vi "SetParam.vi"(8 "error in (no error)":errorcluster caption="entrée d'erreur (pas d'erreur)", 10 "fbeta_score":T1={"beta"=0.0, "labels"=[], "pos_label"={"dtype_pos_label"="int", "pos_label"="1"}, "average"="binary", "sample_weight"=[], "zero_division"={"dtype_zero_division"="str", "zero_division"="warn"}}, 11 "Fbeta_Score.lvclass":refnum<class "Fbeta_Score.lvclass">) -> (0 "error out":errorcluster caption="sortie d'erreur", 3 "Fbeta_Score.lvclass":refnum<class "Fbeta_Score.lvclass">)   [LabVIEW 2020, in "Fbeta_Score.lvclass"]
doc: "Set Parameters"
uses:
  Fbeta_Score.lvclass
  Fbeta_Score.lvclass/Fbeta_Score.ctl
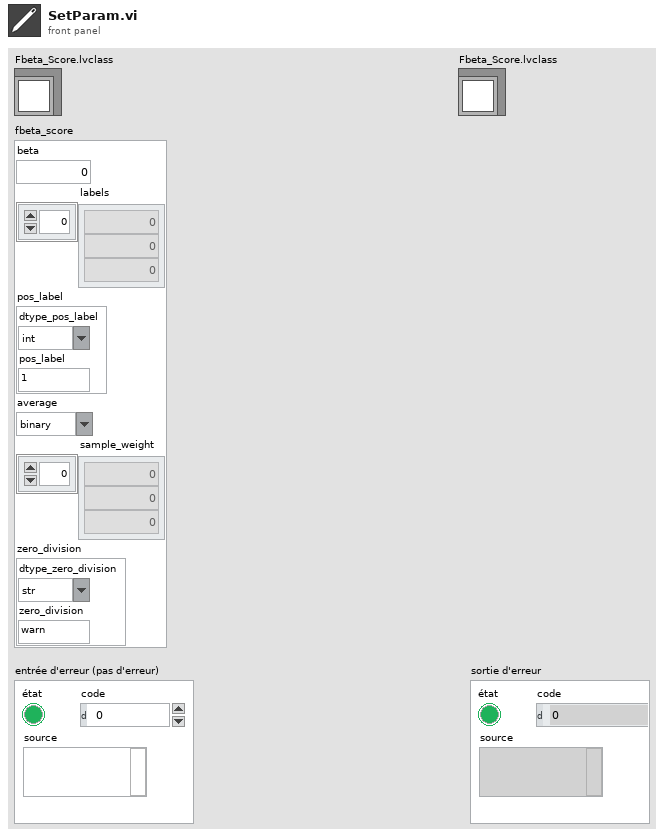
[diagram p1: front panel]
types:
  T1 = cluster{"beta":dbl, "labels":i32[], "pos_label":cluster{"dtype_pos_label":string, "pos_label":string}, "average":string, "sample_weight":dbl[], "zero_division":cluster{"dtype_zero_division":string, "zero_division":string}}
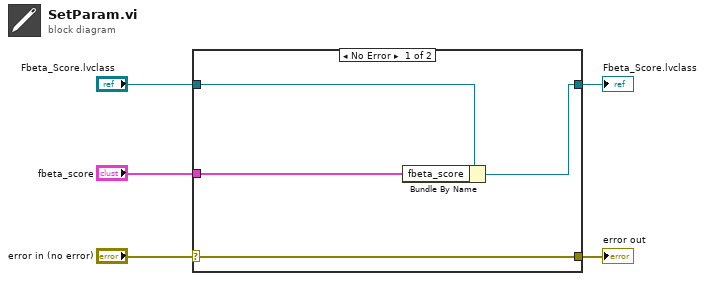
[diagram p0: block diagram]
diagram:
  n1 = case shown="No Error" "error in (no error)" {
    selector: "error in (no error)" -> [w9 w10]
    tunnel: [w9 w10] -> w4
    tunnel: [w7 w11] -> w2
    tunnel: "Fbeta_Score.lvclass" -> [w8 w11]
    tunnel: "fbeta_score" -> [w6 _]
    frame No Error {
      n2 = Bundle By Name(cluster=w8, "fbeta_score"=w6) -> (w7:refnum<class "Fbeta_Score.lvclass">)
    }
    frame Error {
    }
  }
  "error out" <- w4
  "Fbeta_Score.lvclass" <- w2
